vi "Equals.vi"(1 "comparable b":string, 2 "comparable a":string, 3 "Equals Functor":refnum<class "Equal Via Regular Expression Functor.lvclass">) -> (0 "equal?":bool)   [LabVIEW 2023, in "Equal Via Regular Expression Functor.lvclass"]
doc: "Returns whether <b>comparable a</b> is a string that fulfills the regular expression defined by <b>comparable b</b>."
uses:
  Equal Via Regular Expression Functor.lvclass
  <vilib>/regexp/Match Regular Expression.xnode
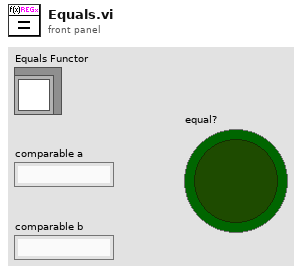
[diagram p1: front panel]
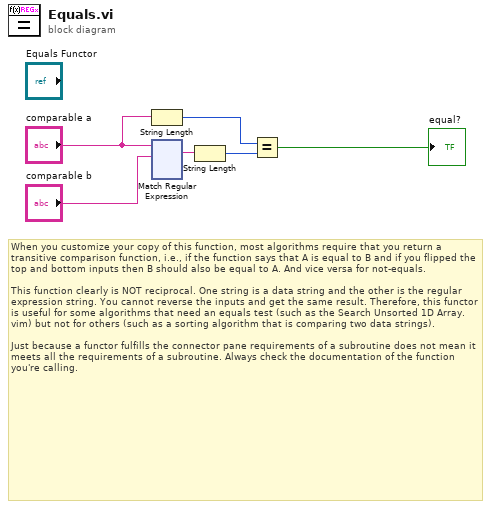
[diagram p0: block diagram]
diagram:
  # "When you customize your copy of this function, most algorithms require that you return a transitive comparison function, i.e., if the function says that A is equal to B and if you flipped the top and bottom inputs then B should also be equal to A. And vice versa for not-equals.\n\nThis function clearly is NOT reciprocal. One string is a data string and the other is the regular expression string. You cannot reverse the inputs and get the same result. Therefore, this functor is useful for some algorithms that need an equals test (such as the Search Unsorted 1D Array.vim) but not for others (such as a sorting algorithm that is comparing two data strings).\n\nJust because a functor fulfills the connector pane requirements of a subroutine does not mean it meets all the requirements of a subroutine. Always check the documentation of the function you're calling."
  n1 = String Length(string="comparable a") -> (length=w4:i32)
  n2 = xnode "Match Regular Expression"("input string"="comparable a", "regular expression"="comparable b") -> ("whole match"=w2:string)  [unwired: 4 in, 4 out]
  n3 = String Length(string=w2) -> (length=w1:i32)
  n4 = Equal?(x=w4, y=w1) -> (x = y?=→"equal?":bool)
